vi "RMGetConfig.vi"(11 "ResultManager":T3) -> (2 "config":T1={"Number of beads"=0, "Number of frame info columns"=0, "Result scaling"={"X"=0.0, "Y"=0.0, "Z"=0.0}, "Result offset"={"X"=0.0, "Y"=0.0, "Z"=0.0}, "Write Interval"=100, "Max frames in memory"=100, "Binary output (1/0)"=0}, 3 "ResultManager (out)":T3)   [LabVIEW 2011]
uses:
  ResultManagerInstance.ctl
  ResultManagerConfig.ctl
  XYZf.ctl
  QTrkDLL.vi
panel:
  out "error out":errorcluster
  in  "error in (no error)":errorcluster
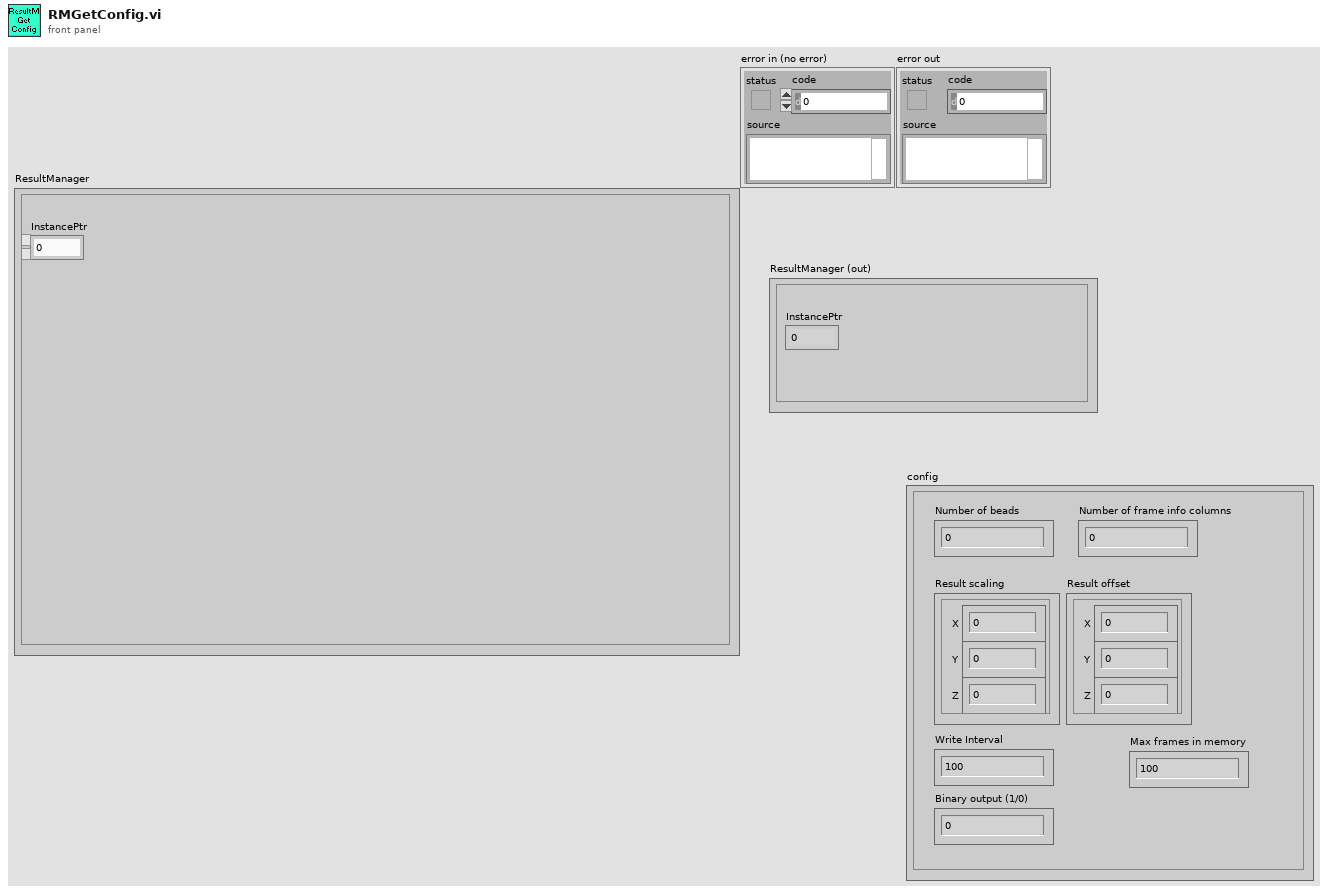
[diagram p1: front panel]
types:
  T1 = typedef "ResultManagerConfig.ctl" = cluster{"Number of beads":i32, "Number of frame info columns":i32, "Result scaling":T2, "Result offset":T2, "Write Interval":i32, "Max frames in memory":i32, "Binary output (1/0)":i8}
  T2 = typedef "XYZf.ctl" = cluster{"X":sgl, "Y":sgl, "Z":sgl}
  T3 = typedef "ResultManagerInstance.ctl" = cluster{"InstancePtr":u64}
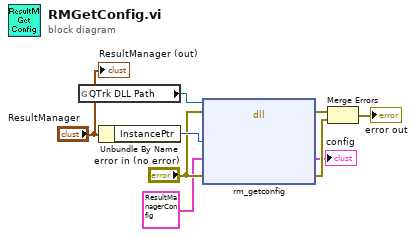
[diagram p0: block diagram]
diagram:
  n1 = global read "QTrkDLL.vi" "QTrk DLL Path"() -> (w9:path)
  n2 = Unbundle By Name("ResultManager") -> ("InstancePtr"=w7:u64)
  n3 = dll-call lib="D:/jcnossen1/cudaqi-tracker/bin/jtrk-labview.dll" fn="rm_getconfig"(path in=w9, error in="error in (no error)", "resultmanager"=w7, "config"=T1 {"Number of beads"=0, "Number of frame info columns"=0, "Result scaling"={"X"=0.0, "Y"=0.0, "Z"=0.0}, "Result offset"={"X"=0.0, "Y"=0.0, "Z"=0.0}, "Write Interval"=100, "Max frames in memory"=100, "Binary output (1/0)"=0} ("ResultManagerConfig"), "error"="error in (no error)") -> (error out=w5:errorcluster, "config"=→"config":T1, "error"=w4:errorcluster)  [unwired: 3 in, 1 out]
  n4 = Merge Errors(w5, w4) -> (→"error out":errorcluster)
  "ResultManager (out)" <- "ResultManager"
